vi "cálculo_joints.vi"(8 "Joint 2":T1(ring), 9 "Joint":T1(ring), 10 "joint 2":dbl[](array[numeric]), 11 "Joint 1":dbl[][](array[numeric])) -> (3 "Array Joints":dbl[](array[numeric]))   [LabVIEW 2016]
panel:
  out "Distância(entre joints)":dbl
  out "Distância ( Produndidade)":dbl
  out "ângulo":dbl
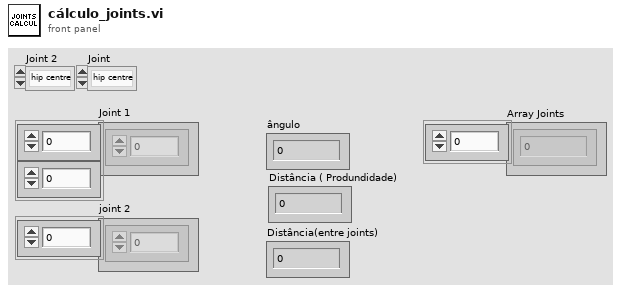
[diagram p1: front panel]
types:
  T1 = enum16{"hip centre", "spine", "shoulder centre", "head", "shoulder left", "elbow left", "wrist left", "hand left", "shoulder right", "elbow right", "wrist right", "hand right", "hip left", "knee left", "ankle left", "foot left", "hip right", "knee right", "ankle right", "foot right"}
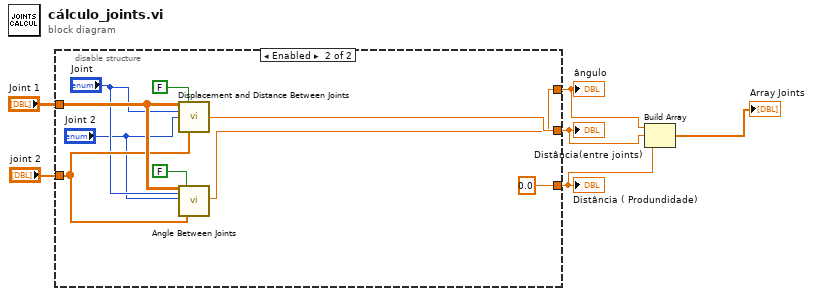
[diagram p0: block diagram]
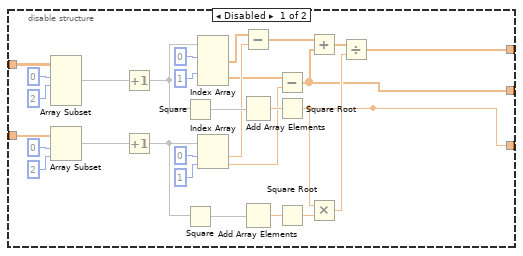
[diagram p2: hidden frame]
diagram:
  n1 = disable-structure shown="Enabled" {
    disable-tunnel: "Joint 1" -> [w35 w42]
    disable-tunnel: "joint 2" -> [w32 w41]
    disable-tunnel: [w11 0.0 ("Distância ( Produndidade)")] -> w2
    disable-tunnel: [w10 w39] -> w4
    disable-tunnel: [w9 w43] -> w3
    frame Disabled {
      n2 = Array Subset(array=w35, index (row)=0 ("index"), length (row)=2 ("length")) -> (w31:dbl[][])  [unwired: 2 in]
      n3 = Array Subset(array=w32, index=0, length=2) -> (w20:dbl[])
      n4 = Increment(x=w31) -> (x+1=w28:dbl[][])
      n5 = Increment(x=w20) -> (x+1=w23:dbl[])
      n6 = Square(x=w28) -> (x^2=w27:dbl[][])
      n7 = Square(x=w23) -> (x^2=w24:dbl[])
      n8 = Index Array(array=w28, index (row) #1=0 ("index"), index (row) #2=1 ("index")) -> (element #1=w19:dbl[], element #2=w17:dbl[])  [unwired: 2 in]
      n9 = Index Array(array=w23, index #1=0 ("index"), index #2=1 ("index")) -> (element #1=w18:dbl, element #2=w16:dbl)
      n10 = Subtract(x=w19, y=w18) -> (x-y=w15:dbl[])
      n11 = Add Array Elements(numeric array=w27) -> (sum=w26:dbl)
      n12 = Add Array Elements(numeric array=w24) -> (sum=w25:dbl)
      n13 = Subtract(x=w17, y=w16) -> (x-y=w9:dbl[])
      n14 = Square Root(x=w26) -> (sqrt(x)=w11:dbl)
      n15 = Square Root(x=w25) -> (sqrt(x)=w14:dbl)
      n16 = Add(x=w15, y=w9) -> (x+y=w13:dbl[])
      n17 = Multiply(x=w11, y=w14) -> (x*y=w12:dbl)
      n18 = Divide(x=w13, y=w12) -> (x/y=w10:dbl[])
    }
    frame Enabled {
      n19 = call <vilib>:"Displacement and Distance Between Joints.vi"("Array of Joint Positions"=w42, "Custom Coordinates Instead of Joint 2"=FALSE, "Joint 1"="Joint", "Joint 2"="Joint 2", "Custom Coordinates"=w41) -> ("Absolute Distance Between Joints"=w43:dbl)  [unwired: 8 in, 2 out]
      n20 = call <vilib>:"Angle Between Joints.vi"("Array of Joint Positions"=w42, "Joint 1"="Joint", "Joint 2"="Joint 2", "Compare Vector 1-2 with User defined Vector"=FALSE, "Custom Vector"=w41) -> ("Angle Between Joints (degrees)"=w39:dbl)  [unwired: 9 in, 5 out]
    }
  }
  "ângulo" <- w4
  "Distância ( Produndidade)" <- w2
  "Distância(entre joints)" <- w3
  n21 = Build Array(w4, w3, w2) -> (→"Array Joints":dbl[])
